vi "Config FGV.vi"(0 "Data":T1, 2 "Operation":enum16{"Get", "Set"}(ring), 11 "error in":errorcluster) -> (4 "Tool Path":path, 6 "Firmware":path[](array[path]), 8 "Images":picture[](array[picture]), 10 "Options":string[](array[string]), 15 "error out":errorcluster)   [LabVIEW 2015]
uses:
  Config.ctl
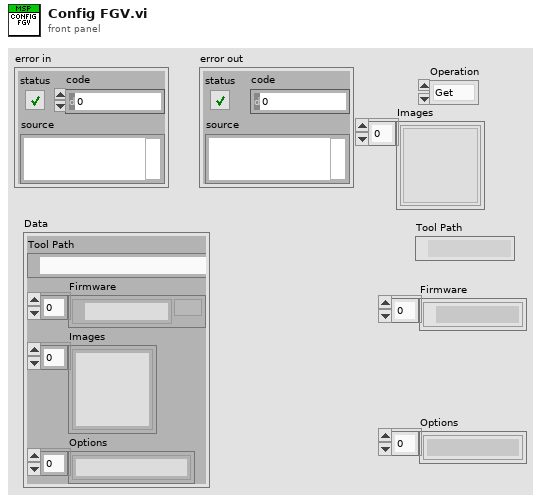
[diagram p1: front panel]
types:
  T1 = typedef "Config.ctl" = cluster{"Tool Path":path, "Firmware":path[], "Images":picture[], "Options":string[]}
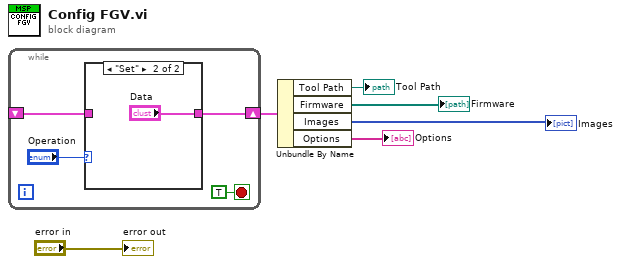
[diagram p0: block diagram]
diagram:
  n1 = while {
    shift-right: [w9] -> w5
    shift-left: _ -> [w8]
    stop <- TRUE stop-if-true
    n2 = case shown="\"Set\"" "Operation" {
      tunnel: [w11 "Data"] -> w9
      tunnel: w8 -> [w11 _]
      frame "Get", Default {
      }
      frame "Set" {
      }
    }
  }
  n3 = Unbundle By Name(w5) -> ("Tool Path"=→"Tool Path":path, "Firmware"=→"Firmware":path[], "Images"=→"Images":picture[], "Options"=→"Options":string[])
  "error out" <- "error in"
